vi "MoAgSy_GPG_readGpgFiles.vi"(0 "MoAgSy_GPG in":refnum<class "MoAgSy_GPG.lvclass">, 1 "options file":path, 2 "keyring file":path, 3 "sec keyring file":path, 5 "error in (no error)":errorcluster, 6 "trust db file":path) -> (11 "Error?":bool[](array[boolean]), 12 "dup trust db file":path, 14 "MoAgSy_GPG out":refnum<class "MoAgSy_GPG.lvclass">, 15 "dup options file":path, 16 "dup keyring file":path, 17 "dup sec keyring file":path, 19 "error out":errorcluster)   [LabVIEW 2009, in "MoAgSy.lvlib" / "MoAgSy_GPG.lvclass"]
uses:
  MoAgSy_GPG.lvclass
  MoAgSy_GPG.lvclass/MoAgSy_GPG.ctl
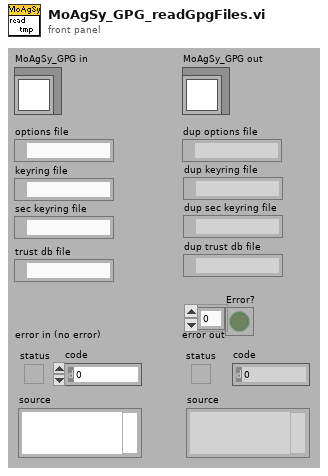
[diagram p1: front panel]
types:
  T1 = cluster{"[0]":string, "[1]":string, "[2]":string, "[3]":string, "[4]":string, "[5]":string, "[6]":string, "[7]":string, "[8]":string}
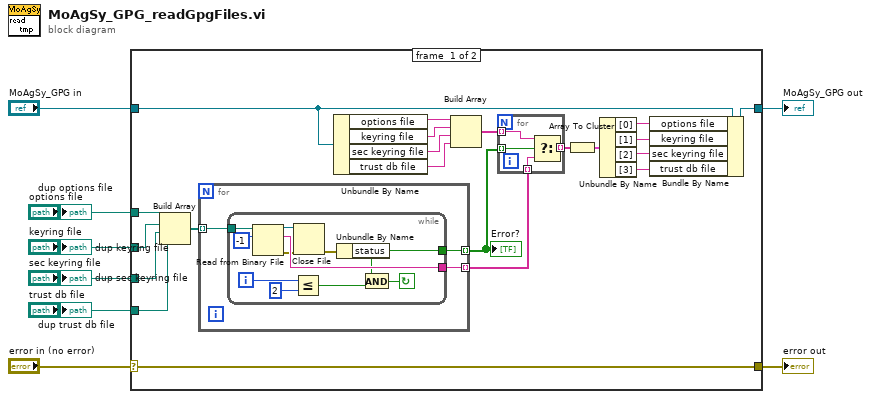
[diagram p0: block diagram]
diagram:
  n1 = case shown="No Error" "error in (no error)" {
    selector: "error in (no error)" -> [w29 w49]
    tunnel: [w29 w49] -> w7
    tunnel: [w22 w48] -> w5
    tunnel: "MoAgSy_GPG in" -> [w23 w48]
    tunnel: "options file" -> [w28 _]
    tunnel: "keyring file" -> [w27 _]
    tunnel: "sec keyring file" -> [w26 _]
    tunnel: "trust db file" -> [w25 _]
    frame #0 {
      n2 = Build Array(w28, w27, w26, w25) -> (w24:path[])
      n3 = for {
        tunnel: w24 -> [w36] mode=indexing
        tunnel: [w35] -> w16 mode=indexing
        tunnel: [w34] -> w9 mode=indexing
        n4 = while {
          tunnel: w36 -> [w46]
          tunnel: [w47] -> w35
          tunnel: [w37] -> w34
          i -> [w41]
          stop <- w39 continue-if-true
          n5 = Read from Binary File(10:-1 ("count (1)"), 11:w46) -> (0:w43:errorcluster, 2:w47:string, 3:w44:refnum<file>)  [unwired: 1 in, 4 out]
          n6 = Less Or Equal?(x=w41, y=2) -> (x <= y?=w38:bool)
          n7 = Close File(refnum=w44, error in=w43) -> (error out=w42:errorcluster)  [unwired: 1 out]
          n8 = Unbundle By Name(w42) -> ("status"=w37:bool)
          n9 = And(x=w37, y=w38) -> (x .and. y?=w39:bool)
        }
      }
      "Error?" <- w9
      n10 = Unbundle By Name(w23) -> ("options file"=w21:string, "keyring file"=w20:string, "sec keyring file"=w19:string, "trust db file"=w18:string)
      n11 = Build Array(w21, w20, w19, w18) -> (w17:string[])
      n12 = for {
        tunnel: w17 -> [w33] mode=indexing
        tunnel: w16 -> [w32] mode=indexing
        tunnel: [w31] -> w15 mode=indexing
        tunnel: w9 -> [w30] mode=indexing
        n13 = Select(t=w33, s=w30, f=w32) -> (s? t:f=w31:string)
      }
      n14 = Array To Cluster(array=w15) -> (cluster=w14:T1)
      n15 = Unbundle By Name(w14) -> ("[0]"=w13:string, "[1]"=w12:string, "[2]"=w11:string, "[3]"=w10:string)
      n16 = Bundle By Name(cluster=w23, "options file"=w13, "keyring file"=w12, "sec keyring file"=w11, "trust db file"=w10) -> (w22:refnum<class "MoAgSy_GPG.lvclass">)
    }
    frame #1 {
    }
  }
  "error out" <- w7
  "MoAgSy_GPG out" <- w5
  "dup options file" <- "options file"
  "dup keyring file" <- "keyring file"
  "dup sec keyring file" <- "sec keyring file"
  "dup trust db file" <- "trust db file"
